vi "Parse qUSG SYS Answer.vi"(0 "Answer To Parse":string, 5 "error in":errorcluster) -> (14 "Function Unit Info List":T1[](array[typedef]), 19 "error out":errorcluster)   [LabVIEW 2026]
doc: "Parse a SPV? structured answer to a array of parameter sets.\nWill return a warning if some parameters could not be parsed."
uses:
  GeneralCommands/UnitDescription.ctl
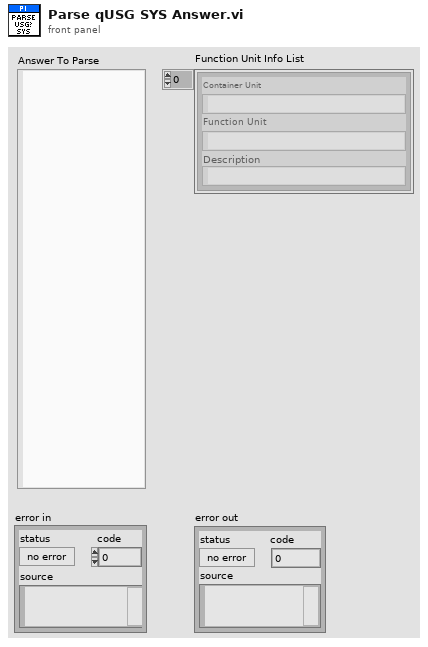
[diagram p1: front panel]
types:
  T1 = typedef "UnitDescription.ctl" = cluster{"Container Unit":string, "Function Unit":string, "Description":string}
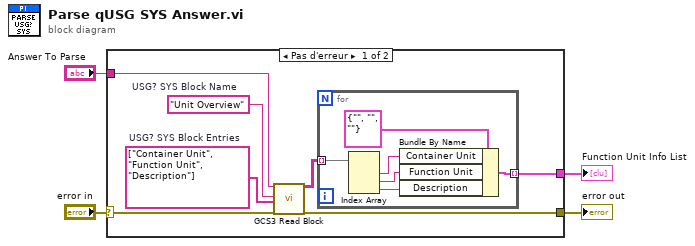
[diagram p0: block diagram]
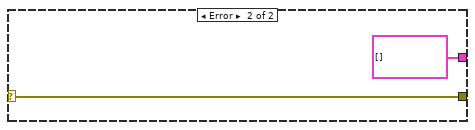
[diagram p2: hidden frame]
diagram:
  n1 = case shown="Pas d'erreur" "error in" {
    selector: "error in" -> [w11 w19]
    tunnel: "Answer To Parse" -> [w10 _]
    tunnel: [w5 T1[] []] -> w1
    tunnel: [w7 w19] -> w2
    frame No Error {
      w8 = string[] ["Container Unit", "Function Unit", "Description"]  # USG? SYS Block Entries
      w9 = "Unit Overview"  # USG? SYS Block Name
      n2 = call "GCS3 Read Block.vi"("GCS 3.0 Block to Parse"=w10, "Expected GCS 3.0 Block Name"=w9, "List of expected GCS 3.0 Block Entries"=w8, "error in"=w11) -> ("List of extracted GCS 3.0 Block Entries"=w6:string[][], "error out"=w7:errorcluster)  [unwired: 14 in]
      n3 = for {
        tunnel: w6 -> [w12] mode=indexing
        tunnel: [w13] -> w5 mode=indexing
        n4 = Index Array(array=w12) -> (element #1=w16:string, element #2=w15:string, element #3=w17:string)  [unwired: 3 in]
        n5 = Bundle By Name(cluster=T1 {"Container Unit"="", "Function Unit"="", "Description"=""} ("Function Unit Info"), "Container Unit"=w16, "Function Unit"=w15, "Description"=w17) -> (w13:T1)
      }
    }
    frame Error {
    }
  }
  "error out" <- w2
  "Function Unit Info List" <- w1
